vi "TestAngleTeleOp.vi"(9 "Send":bool, 10 "Duration":dbl, 11 "Speed":dbl(knob) scale=0.0..1.0 scale format="%#_10g") -> ()   [LabVIEW 2015]
uses:
  Framework/Robot Global Data.vi
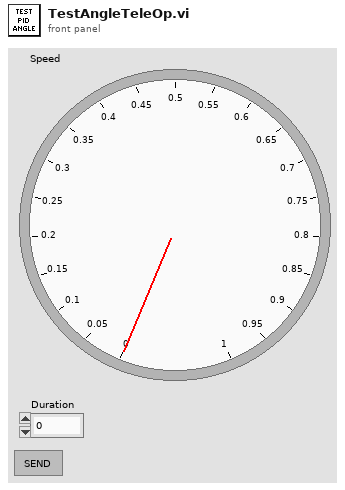
[diagram p1: front panel]
types:
  T1 = typedef "Robot Type Def.ctl" = enum16{"Disabled", "Ghost", "Casper", "Lofty", "Board"}
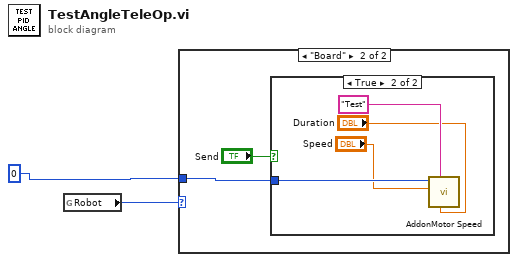
[diagram p0: block diagram]
diagram:
  n1 = global read "Robot Global Data.vi" "Robot"() -> (w2:T1)
  n2 = case shown="\"Board\"" w2 {
    tunnel: 0 -> [_ w4]
    frame "Disabled", Default {
    }
    frame "Board" {
      n3 = case shown="True" "Send" {
        tunnel: w4 -> [_ w7]
        frame False {
        }
        frame True {
          n4 = call "AddonMotor Speed.vi"("Duration"="Duration", "Description"="Test", "Speed"="Speed", "Motor ID"=w7) -> ()  [unwired: 7 in, 1 out]
        }
      }
    }
  }
